vi "Calendar DEMO.vi"() -> ()   [LabVIEW 2020]
uses:
  Calendar Class/DaysOfWeek.ctl
  Calendar Class/Read ColorCalendarBackground.vi
  Calendar Class/Read ColorCalendarSelectionBackground.vi
  Calendar Class/Read ColorCalendarSelectionText.vi
  Calendar Class/Read ColorCalendarText.vi
  Calendar Class/Read ColorDaysOfWeekBackground.vi
  Calendar Class/Read ColorDaysOfWeekText.vi
  Calendar Class/Read ColorSelectorBackground.vi
  Calendar Class/Read ColorSelectorText.vi
  Calendar Class/Read FirstDayOfWeek.vi
  Calendar Class/Read VisibleMonthYearSelect.vi
  Calendar Class/Read VisibleTodaySelector.vi
  Calendar Class/Read VisibleHorizontalLines.vi
  Calendar Class/Read VisibleVerticalLines.vi
  Calendar Class/Read CalendarValue.vi
  Calendar Class/Write ColorSelectorBackground.vi
  Calendar Class/Write ColorDaysOfWeekText.vi
  Calendar Class/Write ColorDaysOfWeekBackground.vi
  Calendar Class/Write ColorSelectorText.vi
  Calendar Class/Write ColorCalendarText.vi
  Calendar Class/Write ColorCalendarBackground.vi
  Calendar Class/Write ColorCalendarSelectionBackground.vi
  Calendar Class/Write ColorCalendarSelectionText.vi
  Calendar Class/Write VisibleTodaySelector.vi
  Calendar Class/Write VisibleMonthYearSelect.vi
  Calendar Class/Write FirstDayOfWeek.vi
  Calendar Class/Write VisibleHorizontalLines.vi
  Calendar Class/Write VisibleVerticalLines.vi
  Calendar Class/Calendar.lvclass
panel:
  in  "Veritcal Lines Visible":bool
  in  "Horizontal Lines Visible":bool
  in  "First Day Of Week":T1
  in  "Month-Year Selector Visible":bool
  in  "Today Selector Visible":bool
  in  "Calendar Selection Text":u32(colorbox)
  in  "Calendar Selection Background":u32(colorbox)
  in  "Calendar Background":u32(colorbox)
  in  "Calendar Text":u32(colorbox)
  in  "Selector Text":u32(colorbox)
  in  "Days of Week Background":u32(colorbox)
  in  "Days of Week Text":u32(colorbox)
  in  "Selector Background":u32(colorbox)
  out "Date Output":timestamp format="%<%A, \n%B %d, %Y>T"
  in  "Calendar":T2={"Calendar"=0, "Month"=0, "Year"=1905, "Today Button"=FALSE, "Previous Month"=FALSE, "Next Month"=FALSE, "Cal Overlay"=FALSE, "Year Selection Underlay"=FALSE} {"Year" min=1600 max=3000; "Month" items=["January", "February", "March", "April", "May", "June", "July", "August", "September", "October", "November", "December"]}
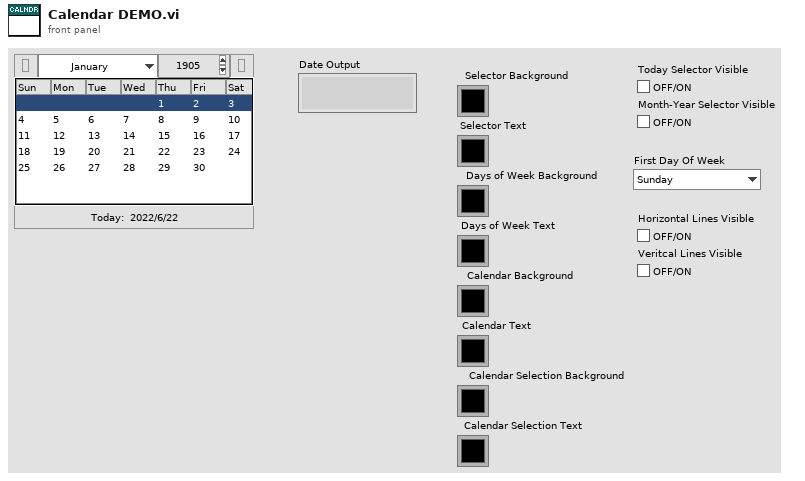
[diagram p1: front panel]
types:
  T1 = typedef "Calendar.lvclass/DaysOfWeek.ctl" = enum16{"Sunday", "Monday", "Tuesday", "Wednesday", "Thursday", "Friday", "Saturday"}
  T2 = cluster{"Calendar":i32, "Month":u16, "Year":i32, "Today Button":bool, "Previous Month":bool, "Next Month":bool, "Cal Overlay":bool, "Year Selection Underlay":bool}
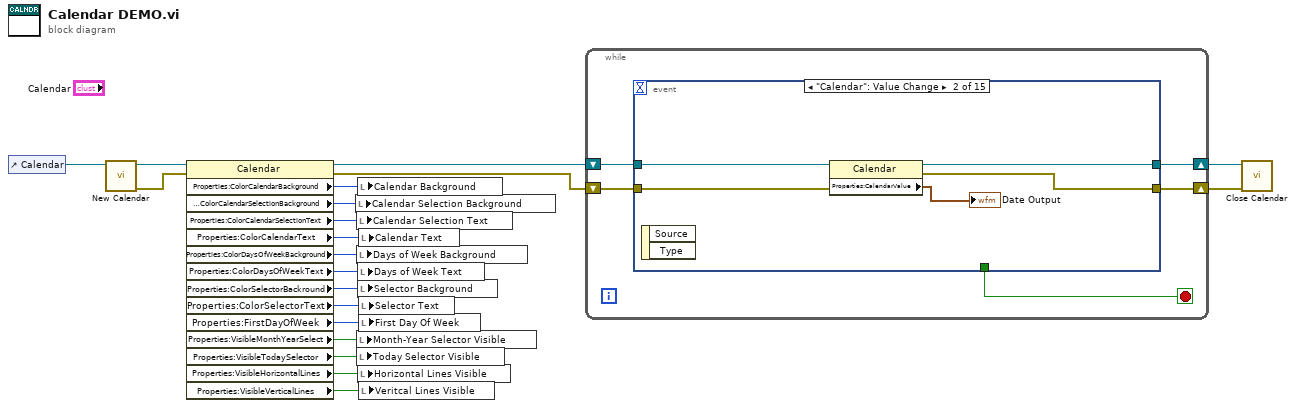
[diagram p0: block diagram]
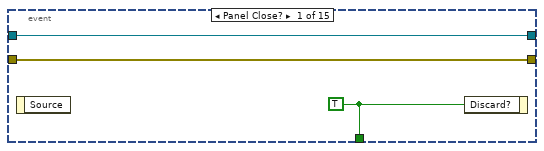
[diagram p2: hidden frame]
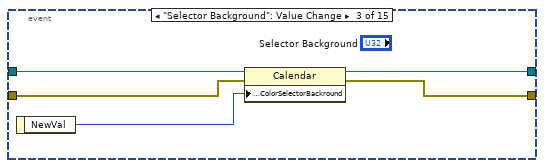
[diagram p3: hidden frame]
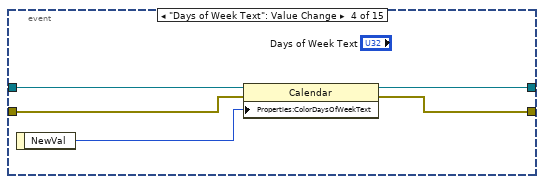
[diagram p4: hidden frame]
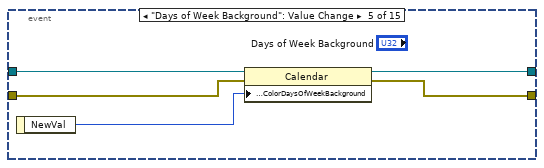
[diagram p5: hidden frame]
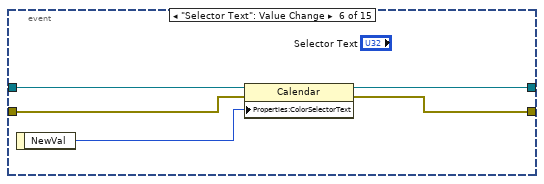
[diagram p6: hidden frame]
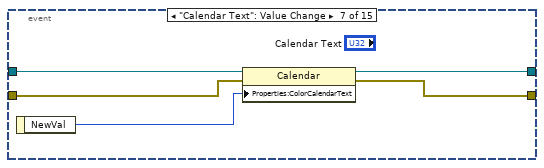
[diagram p7: hidden frame]
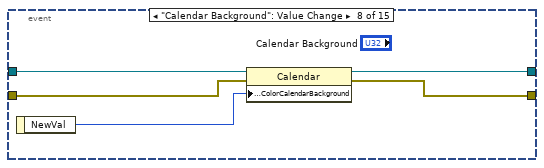
[diagram p8: hidden frame]
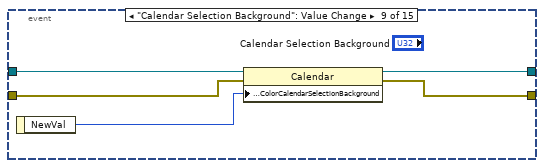
[diagram p9: hidden frame]
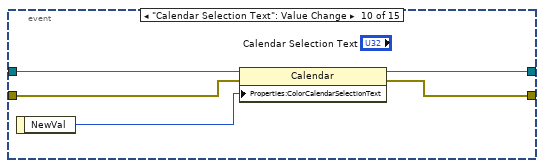
[diagram p10: hidden frame]
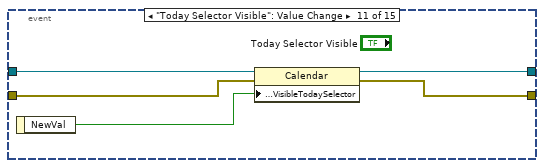
[diagram p11: hidden frame]
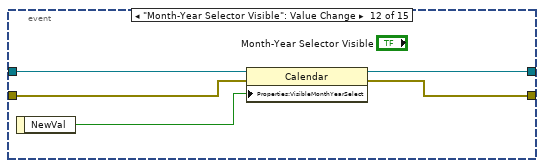
[diagram p12: hidden frame]
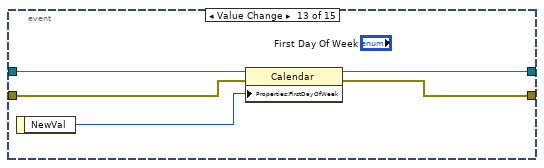
[diagram p13: hidden frame]
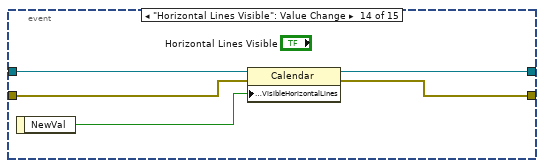
[diagram p14: hidden frame]
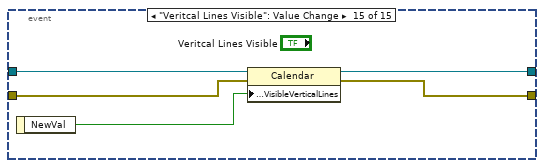
[diagram p15: hidden frame]
diagram:
  n1 = control-ref of="Calendar"() -> (w20:refnum<vi>)
  n2 = call "New Calendar.vi"("Reference"=w20) -> ("error out"=w19:errorcluster, "Calendar out"=w15:refnum<class "Calendar.lvclass">)  [unwired: 8 in, 1 out]
  n3 = property class="Calendar"(reference=w15, error in=w19) -> (reference out=w14:refnum<class "Calendar.lvclass">, error out=w16:errorcluster, "Properties:ColorCalendarBackground"=w13:u32, "Properties:ColorCalendarSelectionBackground"=w12:u32, "Properties:ColorCalendarSelectionText"=w11:u32, "Properties:ColorCalendarText"=w10:u32, "Properties:ColorDaysOfWeekBackground"=w9:u32, "Properties:ColorDaysOfWeekText"=w8:u32, "Properties:ColorSelectorBackround"=w7:u32, "Properties:ColorSelectorText"=w6:u32, "Properties:FirstDayOfWeek"=w5:T1, "Properties:VisibleMonthYearSelect"=w4:bool, "Properties:VisibleTodaySelector"=w3:bool, "Properties:VisibleHorizontalLines"=w2:bool, "Properties:VisibleVerticalLines"=w1:bool)
  n4 = local write "Calendar Selection Background"(w12) -> ()
  n5 = local write "Calendar Selection Text"(w11) -> ()
  n6 = local write "Days of Week Background"(w9) -> ()
  n7 = local write "Month-Year Selector Visible"(w4) -> ()
  n8 = local write "Today Selector Visible"(w3) -> ()
  n9 = local write "Calendar Background"(w13) -> ()
  n10 = local write "Days of Week Text"(w8) -> ()
  n11 = local write "Selector Background"(w7) -> ()
  n12 = local write "Horizontal Lines Visible"(w2) -> ()
  n13 = local write "Calendar Text"(w10) -> ()
  n14 = local write "Selector Text"(w6) -> ()
  n15 = local write "First Day Of Week"(w5) -> ()
  n16 = local write "Veritcal Lines Visible"(w1) -> ()
  n17 = while {
    shift-right: [w24] -> w18
    shift-left: w14 -> [w23]
    shift-right: [w21] -> w17
    shift-left: w16 -> [w22]
    stop <- w25 stop-if-true
    n18 = event shown="[1] \"Calendar\": Value Change" {
      selector: _ -> [_ _ _ _ _ _ _ _ _ _ _ _ _ _ _]
      dyn-events: _ -> [_ _ _ _ _ _ _ _ _ _ _ _ _ _ _]
      timeout: _ -> [_ _ _ _ _ _ _ _ _ _ _ _ _ _ _]
      tunnel: [w28 _ _ _ _ _ _ _ _ _ _ _ _ _ _] -> w25
      tunnel: [w27 w30 w35 w40 w45 w50 w55 w60 w65 w70 w75 w80 w85 w90 w95] -> w24
      tunnel: w23 -> [w27 w33 w38 w43 w48 w53 w58 w63 w68 w73 w78 w83 w88 w93 w98]
      tunnel: w22 -> [w26 w32 w37 w42 w47 w52 w57 w62 w67 w72 w77 w82 w87 w92 w97]
      tunnel: [w26 w29 w34 w39 w44 w49 w54 w59 w64 w69 w74 w79 w84 w89 w94] -> w21
      event Panel Close? {
        w28 = TRUE
        n19 = event-data() -> ()  [unwired: 1 in, 1 out]
        n20 = event-data("Discard?"=w28) -> ()  [unwired: 1 in, 1 out]
      }
      event "Calendar": Value Change {
        n21 = event-data() -> ()  [unwired: 1 in, 2 out]
        n22 = property class="Calendar"(reference=w33, error in=w32) -> (reference out=w30:refnum<class "Calendar.lvclass">, error out=w29:errorcluster, "Properties:CalendarValue"=→"Date Output":timestamp)
      }
      event "Selector Background": Value Change {
        n23 = event-data() -> ("NewVal"=w36:u32)  [unwired: 1 in]
        n24 = property class="Calendar"(reference=w38, error in=w37, "Properties:ColorSelectorBackround"=w36) -> (reference out=w35:refnum<class "Calendar.lvclass">, error out=w34:errorcluster)
      }
      event "Days of Week Text": Value Change {
        n25 = event-data() -> ("NewVal"=w41:u32)  [unwired: 1 in]
        n26 = property class="Calendar"(reference=w43, error in=w42, "Properties:ColorDaysOfWeekText"=w41) -> (reference out=w40:refnum<class "Calendar.lvclass">, error out=w39:errorcluster)
      }
      event "Days of Week Background": Value Change {
        n27 = event-data() -> ("NewVal"=w46:u32)  [unwired: 1 in]
        n28 = property class="Calendar"(reference=w48, error in=w47, "Properties:ColorDaysOfWeekBackground"=w46) -> (reference out=w45:refnum<class "Calendar.lvclass">, error out=w44:errorcluster)
      }
      event "Selector Text": Value Change {
        n29 = event-data() -> ("NewVal"=w51:u32)  [unwired: 1 in]
        n30 = property class="Calendar"(reference=w53, error in=w52, "Properties:ColorSelectorText"=w51) -> (reference out=w50:refnum<class "Calendar.lvclass">, error out=w49:errorcluster)
      }
      event "Calendar Text": Value Change {
        n31 = event-data() -> ("NewVal"=w56:u32)  [unwired: 1 in]
        n32 = property class="Calendar"(reference=w58, error in=w57, "Properties:ColorCalendarText"=w56) -> (reference out=w55:refnum<class "Calendar.lvclass">, error out=w54:errorcluster)
      }
      event "Calendar Background": Value Change {
        n33 = event-data() -> ("NewVal"=w61:u32)  [unwired: 1 in]
        n34 = property class="Calendar"(reference=w63, error in=w62, "Properties:ColorCalendarBackground"=w61) -> (reference out=w60:refnum<class "Calendar.lvclass">, error out=w59:errorcluster)
      }
      event "Calendar Selection Background": Value Change {
        n35 = event-data() -> ("NewVal"=w66:u32)  [unwired: 1 in]
        n36 = property class="Calendar"(reference=w68, error in=w67, "Properties:ColorCalendarSelectionBackground"=w66) -> (reference out=w65:refnum<class "Calendar.lvclass">, error out=w64:errorcluster)
      }
      event "Calendar Selection Text": Value Change {
        n37 = event-data() -> ("NewVal"=w71:u32)  [unwired: 1 in]
        n38 = property class="Calendar"(reference=w73, error in=w72, "Properties:ColorCalendarSelectionText"=w71) -> (reference out=w70:refnum<class "Calendar.lvclass">, error out=w69:errorcluster)
      }
      event "Today Selector Visible": Value Change {
        n39 = event-data() -> ("NewVal"=w76:bool)  [unwired: 1 in]
        n40 = property class="Calendar"(reference=w78, error in=w77, "Properties:VisibleTodaySelector"=w76) -> (reference out=w75:refnum<class "Calendar.lvclass">, error out=w74:errorcluster)
      }
      event "Month-Year Selector Visible": Value Change {
        n41 = event-data() -> ("NewVal"=w81:bool)  [unwired: 1 in]
        n42 = property class="Calendar"(reference=w83, error in=w82, "Properties:VisibleMonthYearSelect"=w81) -> (reference out=w80:refnum<class "Calendar.lvclass">, error out=w79:errorcluster)
      }
      event Value Change {
        n43 = event-data() -> ("NewVal"=w86:T1)  [unwired: 1 in]
        n44 = property class="Calendar"(reference=w88, error in=w87, "Properties:FirstDayOfWeek"=w86) -> (reference out=w85:refnum<class "Calendar.lvclass">, error out=w84:errorcluster)
      }
      event "Horizontal Lines Visible": Value Change {
        n45 = event-data() -> ("NewVal"=w91:bool)  [unwired: 1 in]
        n46 = property class="Calendar"(reference=w93, error in=w92, "Properties:VisibleHorizontalLines"=w91) -> (reference out=w90:refnum<class "Calendar.lvclass">, error out=w89:errorcluster)
      }
      event "Veritcal Lines Visible": Value Change {
        n47 = event-data() -> ("NewVal"=w96:bool)  [unwired: 1 in]
        n48 = property class="Calendar"(reference=w98, error in=w97, "Properties:VisibleVerticalLines"=w96) -> (reference out=w95:refnum<class "Calendar.lvclass">, error out=w94:errorcluster)
      }
    }
  }
  n49 = call "Close Calendar.vi"("error in (no error)"=w17, "Calendar in"=w18) -> ()  [unwired: 9 in, 1 out]
